vi "Call SubPanel Blink.vi"() -> ()   [LabVIEW 2010]
uses:
  Source Code/SubVIs/Front Panel.llb/Operation__FP-BMA.ctl
  Source Code/SubVIs/Front Panel.llb/Warnings__FP-BMA.ctl
  Source Code/SubVIs/Front Panel.llb/Input__FP-BMA.ctl
  Source Code/SubVIs/Front Panel.llb/Output__FP-BMA.ctl
  Source Code/SubVIs/Front Panel.llb/PID Sets__FP-BMA.ctl
  Source Code/SubVIs/Front Panel.llb/Cascade__FP-BMA.ctl
  Source Code/SubVIs/Front Panel.llb/Current Step__FP-BMA.ctl
panel:
  in  "F4 Operation":T8={"operation"=TRUE, "Alarms"=FALSE, "Inputs"=FALSE, "Outputs"=FALSE, "PID Sets"=FALSE, "cascade"=FALSE, "Current Step"=FALSE} caption="F4操作"
  in  "停止":bool
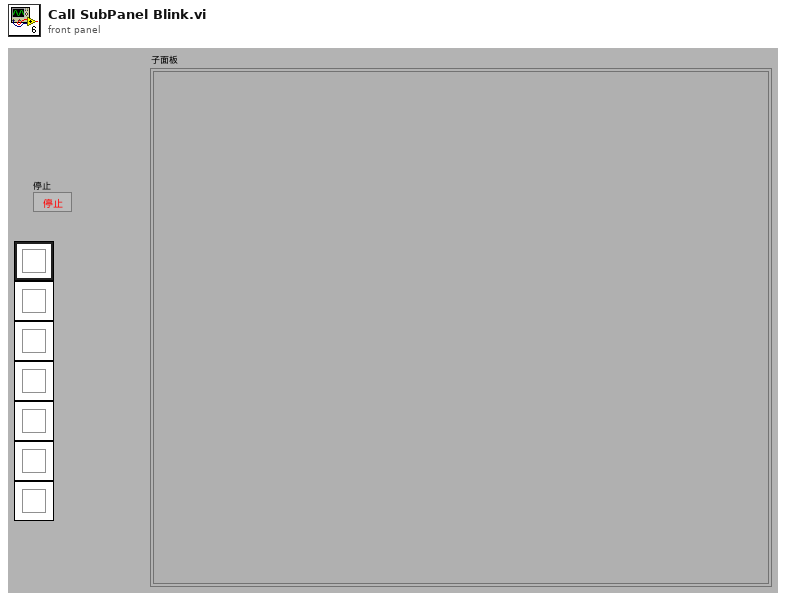
[diagram p1: front panel]
types:
  T1 = typedef "Operation__FP-BMA.ctl" = bool
  T2 = typedef "Warnings__FP-BMA.ctl" = bool
  T3 = typedef "Input__FP-BMA.ctl" = bool
  T4 = typedef "Output__FP-BMA.ctl" = bool
  T5 = typedef "PID Sets__FP-BMA.ctl" = bool
  T6 = typedef "Cascade__FP-BMA.ctl" = bool
  T7 = typedef "Current Step__FP-BMA.ctl" = bool
  T8 = cluster{"operation":T1, "Alarms":T2, "Inputs":T3, "Outputs":T4, "PID Sets":T5, "cascade":T6, "Current Step":T7}
  T9 = cluster{"[0]":bool, "[1]":bool, "[2]":bool, "[3]":bool, "[4]":bool, "[5]":bool, "[6]":bool}
  T10 = typedef "Path InitDynamicVIsPaths__FS.ctl" = cluster{"F4 Operation":path, "F4 Alarms":path, "F4 Inputs":path, "F4 Outputs":path, "F4 PID Sets":path, "F4 Cascade":path, "F4 Current Step":path, "Profile SubPanel":path, "Profile Editor":path, "MainVI":path, "Profile Control":path, "Synergy Control":path, "Driver Server":path}
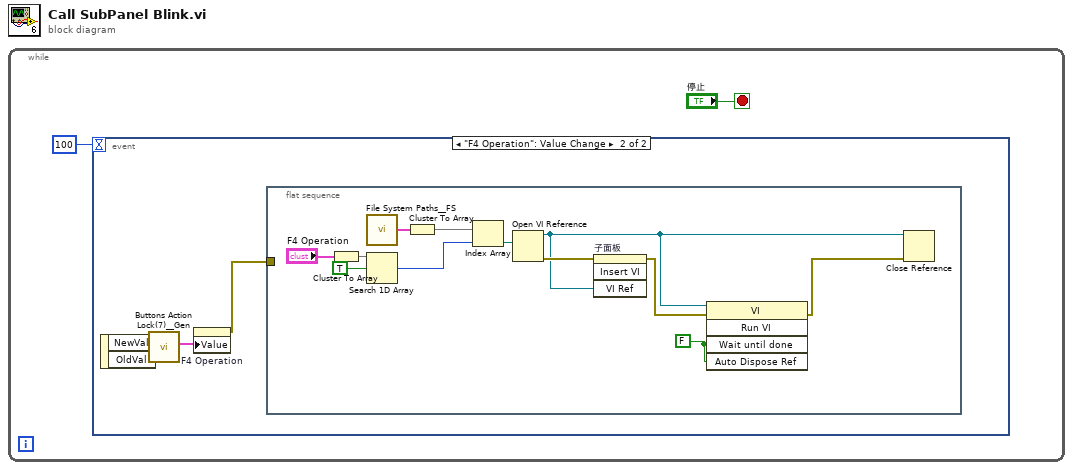
[diagram p0: block diagram]
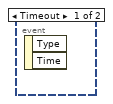
[diagram p2: hidden frame]
diagram:
  n1 = while {
    stop <- "停止" stop-if-true
    n2 = event shown="[1] \"F4 Operation\": Value Change" {
      selector: _ -> [_ _]
      dyn-events: _ -> [_ _]
      timeout: 100 -> [_ _]
      event Timeout {
        n3 = event-data() -> ()  [unwired: 1 in, 2 out]
      }
      event "F4 Operation": Value Change {
        n4 = event-data() -> ("NewVal"=w6:T8, "OldVal"=w5:T8)  [unwired: 1 in]
        n5 = call "Buttons Action Lock(7)__Gen.vi"("Original Value"=w5, "New Value In"=w6) -> ("New Value Out"=w4:T9)  [unwired: 9 in]
        n6 = property on="F4 Operation" class="Clust (strict)"("Value"=w4) -> (error out=w3:errorcluster)  [unwired: 2 in, 1 out]
        n7 = flat-sequence {
          tunnel: w3 -> [_]
          frame #0 {
            w10 = FALSE ("结束前等待")
            n8 = Cluster To Array(cluster="F4 Operation") -> (array=w18:T7[])
            n9 = call "File System Paths__FS.vi"() -> ("DynamicVIs"=w12:T10)  [unwired: 9 in, 2 out]
            n10 = Search 1D Array(1D array=w18, element=T6 TRUE ("元素")) -> (index of element=w15:i32)  [unwired: 1 in]
            n11 = Cluster To Array(cluster=w12) -> (array=w14:path[])
            n12 = Index Array(array=w14, index=w15) -> (element=w16:path)
            n13 = Open VI Reference(vi path=w16) -> (vi reference=w9:refnum<vi>, error out=w11:errorcluster)  [unwired: 5 in]
            n14 = invoke on="子面板" class="子面板" method="Insert VI"(error in=w11, "VI Ref"=w9) -> (error out=w8:errorcluster)  [unwired: 2 in, 3 out]
            n15 = invoke class="VI" method="Run VI"(reference=w9, error in=w8, "Wait until done"=w10, "Auto Dispose Ref"=w10) -> (error out=w7:errorcluster)  [unwired: 1 in, 4 out]
            n16 = Close Reference(reference=w9, error in (no error)=w7) -> ()  [unwired: 1 out]
          }
        }
      }
    }
  }
